vi "CheckOptpump.vi"() -> ()   [LabVIEW 2012]
panel:
  in  "stop":bool
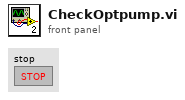
[diagram p1: front panel]
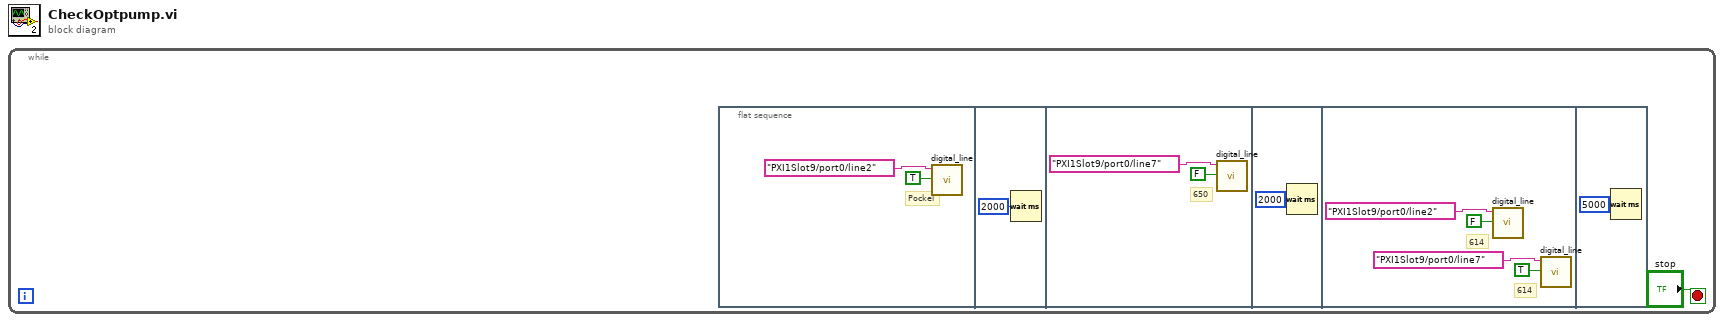
[diagram p0: block diagram]
diagram:
  n1 = while {
    stop <- "stop" stop-if-true
    n2 = flat-sequence {
      frame #0 {
        # "Pockel"
        n3 = call "digital_line.vi"("Boolean"=TRUE, "lines"=tag "PXI1Slot9/port0/line2") -> ()  [unwired: 5 in, 1 out]
      }
      frame #1 {
        n4 = Wait (ms)(milliseconds to wait=u32 2000) -> ()  [unwired: 1 out]
      }
      frame #2 {
        # "650"
        n5 = call "digital_line.vi"("Boolean"=FALSE, "lines"=tag "PXI1Slot9/port0/line7") -> ()  [unwired: 5 in, 1 out]
      }
      frame #3 {
        n6 = Wait (ms)(milliseconds to wait=u32 2000) -> ()  [unwired: 1 out]
      }
      frame #4 {
        # "614"
        # "614"
        n7 = call "digital_line.vi"("Boolean"=FALSE, "lines"=tag "PXI1Slot9/port0/line2") -> ()  [unwired: 5 in, 1 out]
        n8 = call "digital_line.vi"("Boolean"=TRUE, "lines"=tag "PXI1Slot9/port0/line7") -> ()  [unwired: 5 in, 1 out]
      }
      frame #5 {
        n9 = Wait (ms)(milliseconds to wait=u32 5000) -> ()  [unwired: 1 out]
      }
    }
  }
